vi "Plot Object Event.vi"(4 "Plot Action":enum16{"Update", "Remove", "Nothing"}(ring), 6 "Control Ref Queue":T1, 7 "Multiplot Representation In":T4, 8 "error in (no error)":errorcluster, 9 "Object Cluster In":T7, 10 "Actual Transform In":T2, 11 "3D Plot.lvclass in":refnum<class "3D Plot.lvclass">) -> (0 "error out":errorcluster, 1 "Object Cluster Out":T7, 2 "Actual Transform Out":T2, 3 "3D Plot.lvclass out":refnum<class "3D Plot.lvclass">, 5 "Multiplot Representation Out":T4)   [LabVIEW 2017, in "3D Plot.lvclass"]
uses:
  <vilib>/Math Plots/3D Math Plots/3D Plot/3D Plot/3D Plot.lvclass
  <vilib>/Math Plots/3D Math Plots/3D Plot/3D Plot/Typedef/Object Cluster.ctl
  <vilib>/Math Plots/3D Math Plots/3D Plot/3D Plot/Typedef/Multiplot Representation.ctl
  <vilib>/Math Plots/3D Math Plots/3D Plot/3D Plot/Typedef/Plot Representation.ctl
  <vilib>/Math Plots/3D Math Plots/3D Plot/3D Plot/Typedef/Range Clusters.ctl
  <vilib>/Math Plots/3D Math Plots/3D Plot/3D Plot/Typedef/Mesh Data.ctl
  <vilib>/Math Plots/3D Math Plots/3D Plot/3D Plot/Typedef/Actual Transform.ctl
  <vilib>/Math Plots/3D Math Plots/3D Plot/Action String/3DMathPlot Ctrl Act Queue.ctl
  <vilib>/Math Plots/3D Math Plots/3D Plot/Action String/3DMathPlot Ctrl Act Cluster.ctl
  <vilib>/Math Plots/3D Math Plots/3D Plot/Action String/3DMathPlot State Class.ctl
  <vilib>/picture/3D Picture Control/Object/Create Object (name).vi
  <vilib>/picture/3D Picture Control/NI_3D Picture Control.lvlib
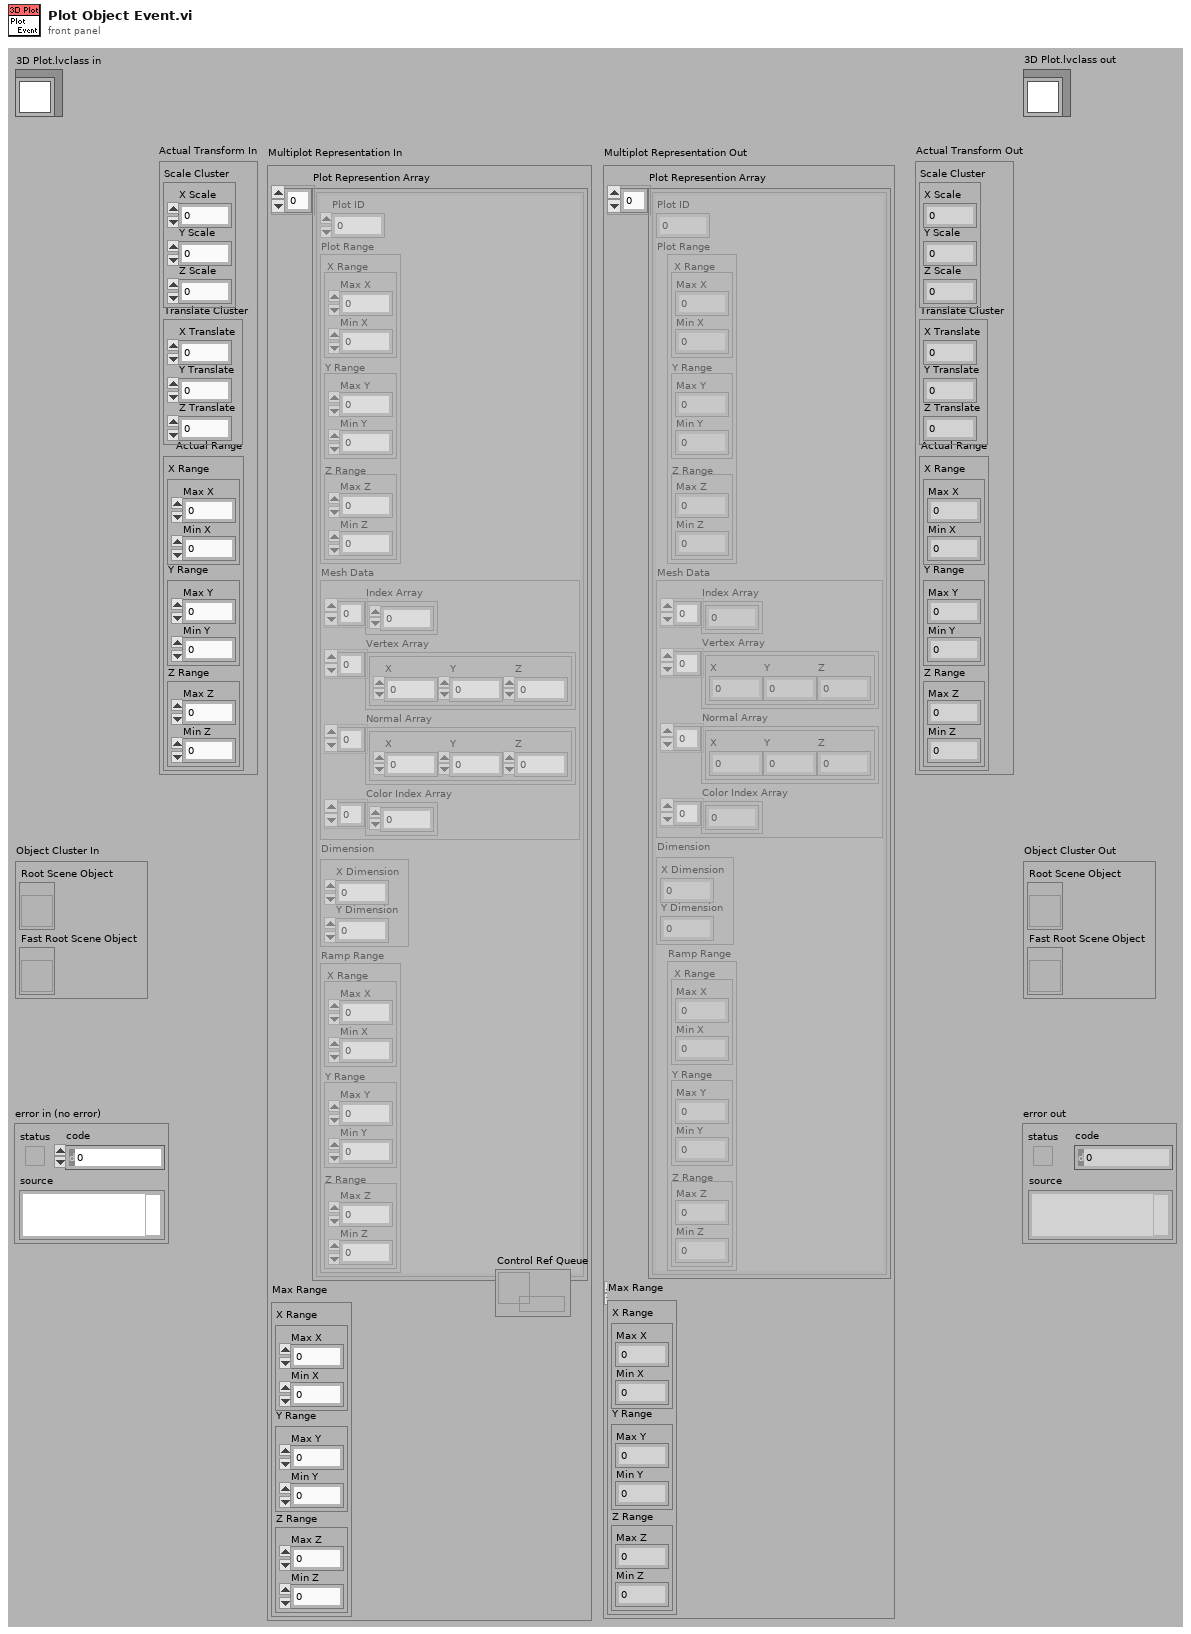
[diagram p1: front panel]
types:
  T1 = typedef "3DMathPlot Ctrl Act Queue.ctl" = refnum<queue>
  T2 = typedef "3D Plot.lvclass/Actual Transform.ctl" = cluster{"Scale Cluster":cluster{"X Scale":sgl, "Y Scale":sgl, "Z Scale":sgl}, "Translate Cluster":cluster{"X Translate":sgl, "Y Translate":sgl, "Z Translate":sgl}, "Actual Range":T3}
  T3 = typedef "3D Plot.lvclass/Range Clusters.ctl" = cluster{"X Range":cluster{"Max X":sgl, "Min X":sgl}, "Y Range":cluster{"Max Y":sgl, "Min Y":sgl}, "Z Range":cluster{"Max Z":sgl, "Min Z":sgl}}
  T4 = typedef "3D Plot.lvclass/Multiplot Representation.ctl" = cluster{"Plot Represention Array":T5[], "Max Range":T3}
  T5 = typedef "3D Plot.lvclass/Plot Representation.ctl" = cluster{"Plot ID":i32, "Plot Range":T3, "Mesh Data":T6, "Dimension":cluster{"X Dimension":i32, "Y Dimension":i32}, "Ramp Range":T3}
  T6 = typedef "3D Plot.lvclass/Mesh Data.ctl" = cluster{"Index Array":u32[], "Vertex Array":cluster{"X":sgl, "Y":sgl, "Z":sgl}[], "Normal Array":cluster{"X":sgl, "Y":sgl, "Z":sgl}[], "Color Index Array":i32[]}
  T7 = typedef "3D Plot.lvclass/Object Cluster.ctl" = cluster{"Root Scene Object":refnum<vi>, "Fast Root Scene Object":refnum<vi>}
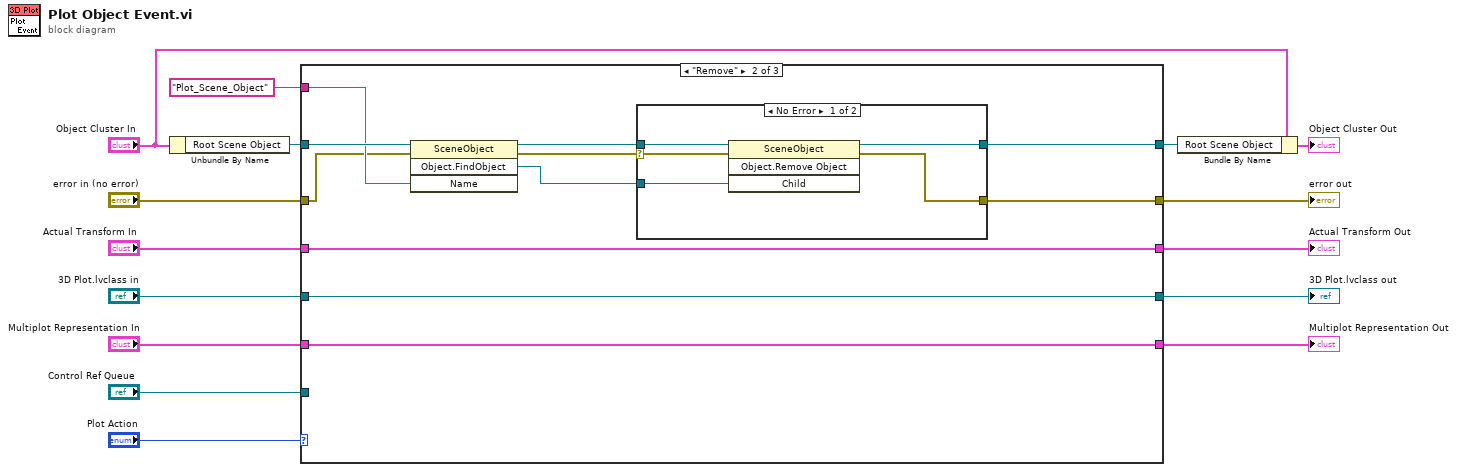
[diagram p0: block diagram]
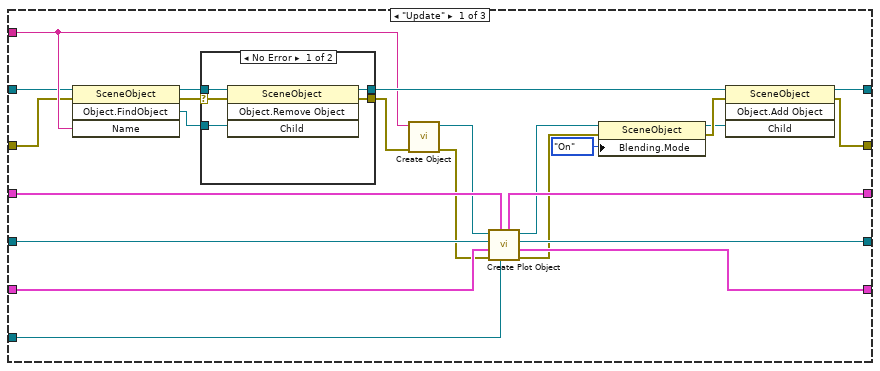
[diagram p2: hidden frame]
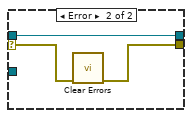
[diagram p3: hidden frame]
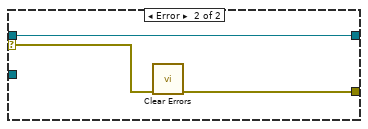
[diagram p4: hidden frame]
diagram:
  n1 = Unbundle By Name("Object Cluster In") -> ("Root Scene Object"=w4:refnum<vi>)
  n2 = case shown="\"Remove\"" "Plot Action" {
    tunnel: "error in (no error)" -> [w17 w49 w71]
    tunnel: [w23 w56 w71] -> w13
    tunnel: "3D Plot.lvclass in" -> [w39 w58 w70]
    tunnel: [w38 w58 w70] -> w12
    tunnel: "Multiplot Representation In" -> [w37 w57 w69]
    tunnel: [w36 w57 w69] -> w9
    tunnel: "Actual Transform In" -> [w35 w55 w68]
    tunnel: [w34 w55 w68] -> w7
    tunnel: w4 -> [w27 w54 w67]
    tunnel: [w22 w50 w67] -> w2
    tunnel: "Control Ref Queue" -> [w33 _ _]
    tunnel: "Plot_Scene_Object" ("Name") -> [w28 w51 _]
    frame "Update" {
      n3 = invoke class="SceneObject" method="Object.FindObject"(reference=w27, error in=w17, "Name"=w28) -> (reference out=w30:refnum<vi>, error out=w16:errorcluster, "FindObject"=w29:refnum<vi>)  [unwired: 1 in, 1 out]
      n4 = case shown="No Error" w16 {
        selector: w16 -> [w40 w46]
        tunnel: [w42 w45] -> w31
        tunnel: w30 -> [w44 w47]
        tunnel: w29 -> [w43 _]
        tunnel: [w41 w47] -> w32
        frame No Error {
          n5 = invoke class="SceneObject" method="Object.Remove Object"(reference=w44, error in=w40, "Child"=w43) -> (reference out=w41:refnum<vi>, error out=w42:errorcluster)  [unwired: 1 in, 2 out]
        }
        frame Error {
          n6 = call <vilib>:"Clear Errors.vi"("error in (no error)"=w46) -> ("error out"=w45:errorcluster)  [unwired: 5 in, 1 out]
        }
      }
      n7 = call-poly <vilib>:"Create Object.vi"("error in (no error)"=w31, "Name"=w28) -> ("error out"=w25:errorcluster, "Scene:New Object"=w26:refnum<vi>)  [unwired: 8 in]
      n8 = call-dynamic "Create Plot Object.vi"("Control Ref Queue"=w33, "Actual Transform In"=w35, "error in (no error)"=w25, "Multiplot Representation In"=w37, "3D Plot.lvclass in"=w39, "Plot Object In"=w26) -> ("error out"=w20:errorcluster, "Multiplot Representation Out"=w36:T4, "3D Plot.lvclass out"=w38:refnum<class "3D Plot.lvclass">, "Plot Object Out"=w24:refnum<vi>, "Actual Transform Out"=w34:T2)  [unwired: 1 out]
      n9 = property class="SceneObject"(reference=w24, error in=w20, "Blending.Mode"=enum16{"Inherit Value", "Off", "On"}."On" ("Blending:Mode")) -> (reference out=w18:refnum<vi>, error out=w19:errorcluster)
      n10 = invoke class="SceneObject" method="Object.Add Object"(reference=w32, error in=w19, "Child"=w18) -> (reference out=w22:refnum<vi>, error out=w23:errorcluster)  [unwired: 1 in, 2 out]
    }
    frame "Remove" {
      n11 = invoke class="SceneObject" method="Object.FindObject"(reference=w54, error in=w49, "Name"=w51) -> (reference out=w53:refnum<vi>, error out=w48:errorcluster, "FindObject"=w52:refnum<vi>)  [unwired: 1 in, 1 out]
      n12 = case shown="No Error" w48 {
        selector: w48 -> [w59 w65]
        tunnel: w52 -> [w63 _]
        tunnel: w53 -> [w62 w66]
        tunnel: [w61 w66] -> w50
        tunnel: [w60 w64] -> w56
        frame No Error {
          n13 = invoke class="SceneObject" method="Object.Remove Object"(reference=w62, error in=w59, "Child"=w63) -> (reference out=w61:refnum<vi>, error out=w60:errorcluster)  [unwired: 1 in, 2 out]
        }
        frame Error {
          n14 = call <vilib>:"Clear Errors.vi"("error in (no error)"=w65) -> ("error out"=w64:errorcluster)  [unwired: 5 in, 1 out]
        }
      }
    }
    frame "Nothing", Default {
    }
  }
  "error out" <- w13
  "3D Plot.lvclass out" <- w12
  "Multiplot Representation Out" <- w9
  "Actual Transform Out" <- w7
  n15 = Bundle By Name(cluster="Object Cluster In", "Root Scene Object"=w2) -> (→"Object Cluster Out":T7)
